vi "AMX-CCD 自动处理图像.vi"(0 "Image In":T1(plugin-control), 11 "error in (no error)":errorcluster caption="错误输入（无错误）") -> (4 "Image Out":T1(plugin-control), 6 "NO LINES":bool, 8 "CCD1-R":bool, 10 "CCD1-L":bool, 15 "error out":errorcluster caption="错误输出")   [LabVIEW 2017]
uses:
  Global System.vi
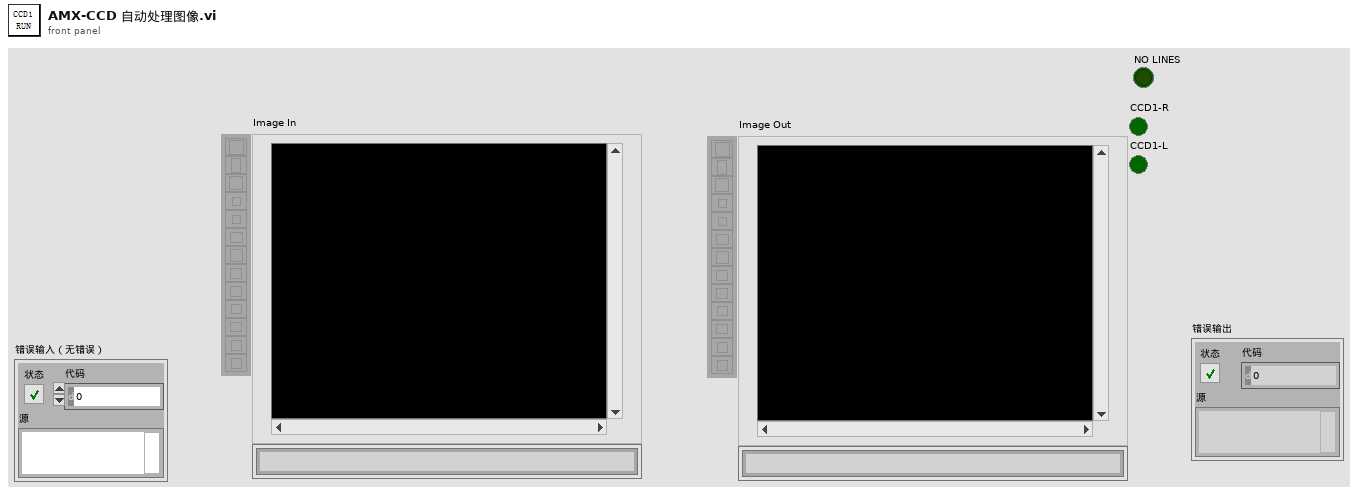
[diagram p1: front panel]
types:
  T1 = typedef "IMAQ Image.ctl" = refnum<image>
  T2 = typedef "IMAQ Rectangle" = cluster{"Left":i32, "Top":i32, "Right":i32, "Bottom":i32, "Rotation":dbl}
  T3 = typedef "IMAQ Line" = cluster{"Start X":i32, "Start Y":i32, "End X":i32, "End Y":i32}
  T4 = cluster{"Rectangle big CCD1":T2, "Rectangle top CCD1 ":T2, "Line":T3, "left line ":dbl, "right line":dbl}
  T5 = typedef "IMAQ Curve Parameters.ctl" = cluster{"Extraction Mode":u32, "Edge Threshold":i32, "Edge Filter Size":u32, "Min Length":i32, "Row Search Step Size":i32, "Col Search Step Size":i32, "Max Endpoint Gap":i32, "Closed":bool, "Subpixel":bool}
  T6 = cluster{"Rectangle":T2, "Angle (degrees) ":sgl, "long":sgl, "abgek":dbl, "Color":u32, "left threshold":dbl, "Rectangle right":T2, "long right":sgl, "abgek right":dbl, "Color 2":u32, "right threshold":dbl, "left":dbl, "right":dbl, "Settings (Big)":T5, "Clamp Settings (Big)":cluster{"Angle ":dbl, "Edge Polarity":cluster{"Start":u32, "End":u32}}, " Settings top":T5, "Clamp Settings top ":cluster{"Angle ":dbl, "Edge Polarity":cluster{"Start":u32, "End":u32}}, "Sub-Pixel Accuracy ":bool, "Threshold Parameters":cluster{"Level Type":enum32{"Absolute Value", "Relative value"}, "Threshold Level":i32, "Hysteresis":i32}, "Process ":enum16{"Get First Edge", "Get First + Last Edge", "Get All Edges"}, "Threshold Parameters 2":cluster{"Level Type":enum32{"Absolute Value", "Relative value"}, "Threshold Level":i32, "Hysteresis":i32}}
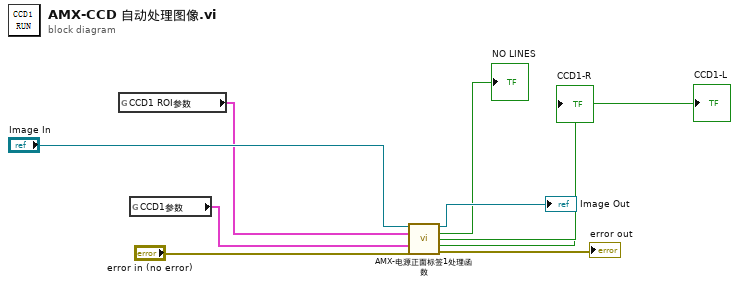
[diagram p0: block diagram]
diagram:
  n1 = global read "Global System.vi" "CCD1 ROI参数"() -> (w1:T4)
  n2 = global read "Global System.vi" "CCD1参数"() -> (w7:T6)
  n3 = call "AMX-电源正面标签1处理函数.vi"("Image in"="Image In", "ROI参数"=w1, "CCD1参数"=w7, "error in (no error)"="error in (no error)") -> ("Image out"=→"Image Out":T1, "NO LINES"=→"NO LINES":bool, "CCD1-R"=→"CCD1-R":bool, "CCD1-L"=→"CCD1-L":bool, "error out"=→"error out":errorcluster)  [unwired: 7 in]
